vi "Send.vi"(5 "Record Topic Name?":bool, 7 "Message Priority":T1, 8 "error in (no error)":errorcluster, 9 "Timeout":i32, 10 "Message":refnum<class "Message Interface.lvclass">, 11 "Message Transport Actor Framework in":refnum<class "Message Transport Actor Framework.lvclass">) -> (0 "error out":errorcluster, 2 "Timed Out?":bool, 3 "Message Transport Actor Framework out":refnum<class "Message Transport Actor Framework.lvclass">)   [LabVIEW 2016, in "Stream Mediator.lvlib" / "Message Transport Actor Framework.lvclass"]
doc: "--\nCopyright © 2017 Composed SystemsI All rights reserved.\n\nAuthor: Jon McBee <jon.mcbee@composed.io>\n\nThis library is provided \"AS IS\" ,WITHOUT WARRANTIES OR\nCONDITIONS OF ANY KIND, either express or implied.\n\nComposed Systems -- composed.io\n\nStream 0.0.1.1\nJon McBee - Composed Systems\nCopyright (c) 2017, Composed Systems"
uses:
  <userlib>/Composed Systems/Stream/Mediator/Classes/Message Transport Actor Framework/Message Transport Actor Framework.lvclass
  C:/Program Files (x86)/National Instruments/LabVIEW 2016/user.lib/Composed Systems/Stream/Mediator/Classes/Message Transport Interface/Message Transport Interface.lvclass
  <userlib>/Composed Systems/Stream/Mediator/Classes/Message Interface/Message Interface.lvclass
  <userlib>/Composed Systems/Stream/Mediator/Classes/Message Transport Interface/Message Priority.ctl
  <userlib>/Composed Systems/Stream/Mediator/Classes/Message Interface/Message Interface.lvclass/Message Interface.ctl
  <userlib>/Composed Systems/Stream/Mediator/Classes/Message Transport Actor Framework/Message Transport Actor Framework.lvclass/Message Transport Actor Framework.ctl
  <vilib>/ActorFramework/Message Enqueuer/Message Priority.ctl
  <userlib>/Composed Systems/Stream/Mediator/Classes/Message AF Mediator/Message AF Mediator.lvclass
  C:/Program Files (x86)/National Instruments/LabVIEW 2016/user.lib/Composed Systems/Stream/Mediator/Classes/Message AF Low Coupling/Message AF Low Coupling.lvclass
  <userlib>/Composed Systems/Stream/Mediator/Classes/Message AF Low Coupling/Message AF Low Coupling.lvclass
  <vilib>/ActorFramework/Message Enqueuer/Message Enqueuer.lvclass
  <userlib>/Composed Systems/Stream/Mediator/Classes/Message Transport Interface/Message Transport Interface.lvclass
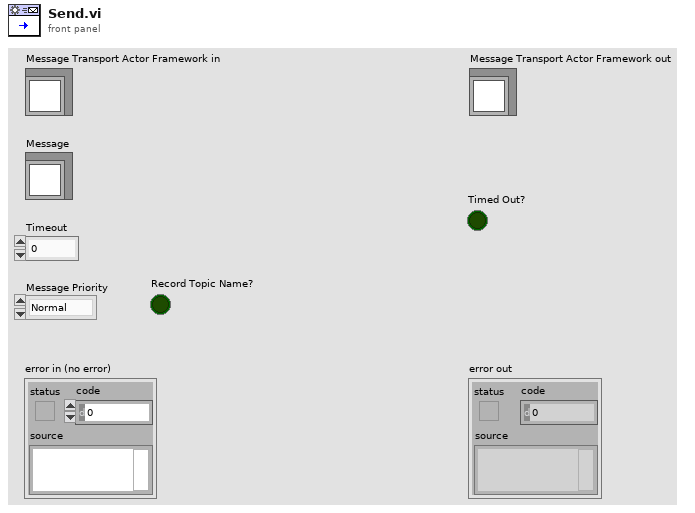
[diagram p1: front panel]
types:
  T1 = typedef "Stream Mediator.lvlib/Message Transport Interface.lvclass/Message Priority.ctl" = enum16{"Normal", "High"}
  T2 = typedef "Actor Framework.lvlib/Message Enqueuer.lvclass/Message Priority.ctl" = enum16{"Low", "Normal", "High"}
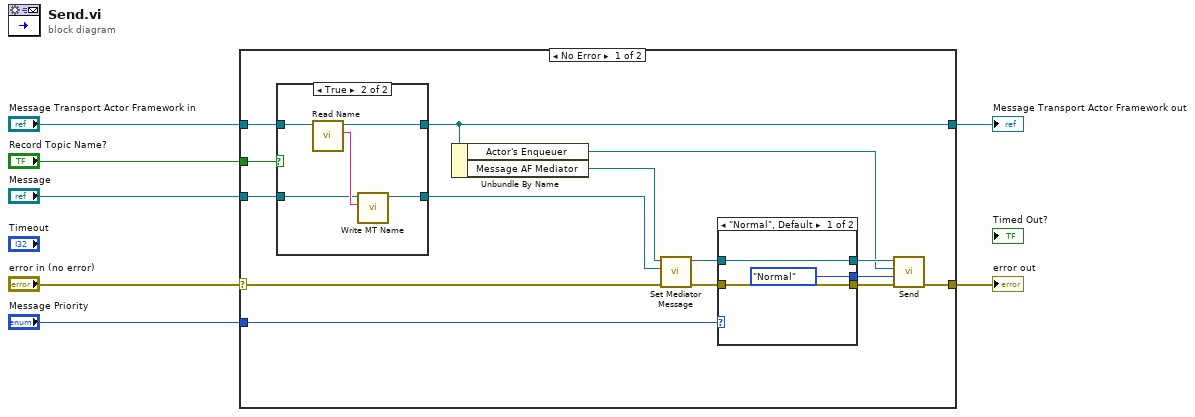
[diagram p0: block diagram]
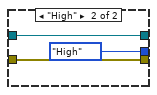
[diagram p3: hidden frame]
diagram:
  n1 = case shown="No Error" "error in (no error)" {
    selector: "error in (no error)" -> [w21 w37]
    tunnel: "Message" -> [w10 _]
    tunnel: [w18 w37] -> w5
    tunnel: [w11 w36] -> w4
    tunnel: "Message Transport Actor Framework in" -> [w12 w36]
    tunnel: "Message Priority" -> [w19 _]
    tunnel: "Record Topic Name?" -> [w8 _]
    frame No Error {
      n2 = case shown="True" w8 {
        tunnel: w12 -> [w24 w28]
        tunnel: [w24 w27] -> w11
        tunnel: w10 -> [w23 w26]
        tunnel: [w23 w25] -> w9
        frame False {
        }
        frame True {
          n3 = call <userlib>:"Read Name.vi"("Message Transport Interface in"=w28) -> ("Name"=w29:string, "Message Transport Interface out"=w27:refnum<class "Message Transport Actor Framework.lvclass">)  [unwired: 8 in, 1 out]
          n4 = call <userlib>:"Write MT Name.vi"("MT Name"=w29, "Message Interface in"=w26) -> ("Message Interface out"=w25:refnum<class "Message Interface.lvclass">)  [unwired: 9 in]
        }
      }
      n5 = Unbundle By Name(w11) -> ("Actor's Enqueuer"=w14:refnum<class "Message Enqueuer.lvclass">, "Message AF Mediator"=w13:refnum<class "Message AF Mediator.lvclass">)
      n6 = call <userlib>:"Set Mediator Message.vi"("error in (no error)"=w21, "Mediator Message"=w9, "Message AF Mediator in"=w13) -> ("error out"=w20:errorcluster, "Message AF Mediator out"=w22:refnum<class "Message AF Mediator.lvclass">)  [unwired: 7 in]
      n7 = case shown="\"Normal\", Default" w19 {
        tunnel: w22 -> [w31 w34]
        tunnel: w20 -> [w32 w35]
        tunnel: [w32 w35] -> w17
        tunnel: [w31 w34] -> w16
        tunnel: [Message_Priority."Normal" ("Message Priority (Normal)") Message_Priority."High" ("Message Priority (Normal)")] -> w15
        frame "Normal", Default {
        }
        frame "High" {
        }
      }
      n8 = call <userlib>:"Send.vi"("error in (no error)"=w17, "Message Priority (Normal)"=w15, "Message Enqueuer in"=w14, "Message AF Low Coupling in"=w16) -> ("error out"=w18:errorcluster)  [unwired: 7 in]
    }
    frame Error {
    }
  }
  "error out" <- w5
  "Message Transport Actor Framework out" <- w4
